vi "AWG Write Butterfly Ramps for 1Channel.vi"(6 "Secondary Pin Name":string, 7 "Main Pin Name":string, 8 "error in (no error)":errorcluster, 9 "AmpGain":dbl, 10 "Voltages":dbl[](array[numeric]), 11 "Automation Refnum in":T1) -> (0 "error out":errorcluster)   [LabVIEW 2013]
uses:
  <vilib>/NI_TestStand_SemiconductorModule/NI_TestStand_Semiconductor_Module.lvlibp/PinMap/General/SemiconductorModuleContext.ctl
  Utility/PreciseRampWaveformWithName.ctl
  Utility/PreciseRampWaveform.ctl
  <vilib>/NI_TestStand_SemiconductorModule/NI_TestStand_Semiconductor_Module.lvlibp
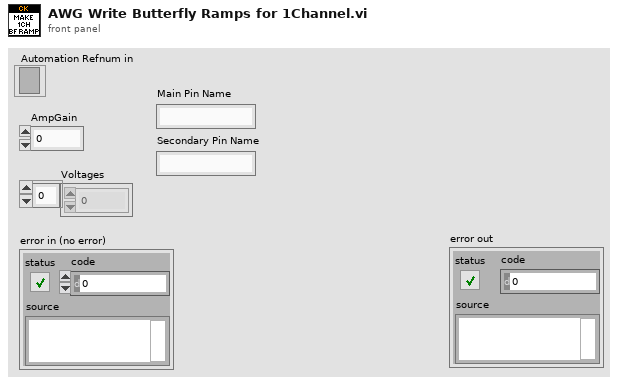
[diagram p1: front panel]
types:
  T1 = typedef "NI_TestStand_Semiconductor_Module.lvlibp/SemiconductorModuleContext.ctl" = refnum<k7>
  T2 = typedef "PreciseRampWaveformWithName.ctl" = cluster{"Name":string, "Waveform":T3}
  T3 = typedef "PreciseRampWaveform.ctl" = cluster{"Start":dbl, "End":dbl, "Time":dbl}
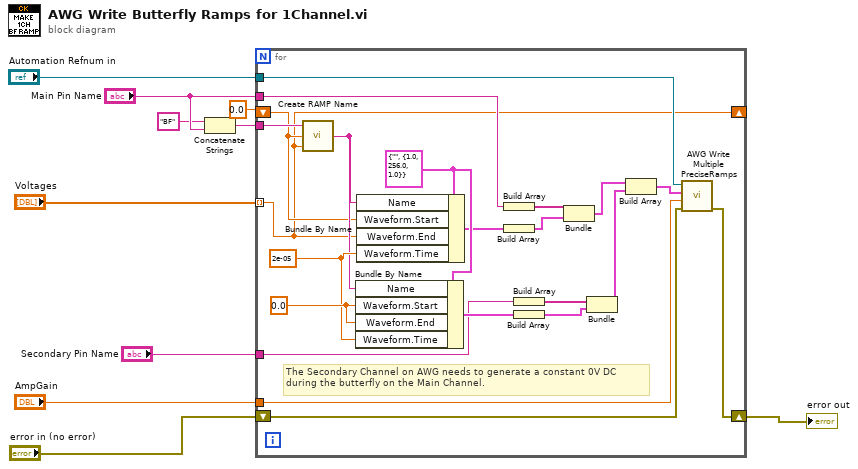
[diagram p0: block diagram]
diagram:
  n1 = Concatenate Strings("BF" ("string"), "Main Pin Name") -> (w5:string)
  n2 = for {
    tunnel: "Voltages" -> [w11] mode=indexing
    tunnel: "Automation Refnum in" -> [w32]
    tunnel: "AmpGain" -> [w30]
    shift-right: [w11] -> _
    shift-left: 0.0 ("Numeric") -> [w12]
    tunnel: "Main Pin Name" -> [w16]
    tunnel: "Secondary Pin Name" -> [w15]
    shift-right: [w14] -> w6
    shift-left: "error in (no error)" -> [w31]
    tunnel: w5 -> [w13]
    w27 = 0.0 ("Start")
    w26 = 2e-05 ("Time")
    w28 = T2 {"Name"="", "Waveform"={"Start"=1.0, "End"=256.0, "Time"=1.0}} ("Waveform In")
    # "The Secondary Channel on AWG needs to generate a constant 0V DC\nduring the butterfly on the Main Channel."
    n3 = call "Create RAMP Name.vi"("Numeric 2"=w11, "Numeric 1"=w12, "Prefix"=w13) -> ("concatenated string"=w23:string)
    n4 = Bundle By Name(cluster=w28, "Name"=w23, "Waveform.Start"=w27, "Waveform.End"=w27, "Waveform.Time"=w26) -> (w24:T2)
    n5 = Bundle By Name(cluster=w28, "Name"=w23, "Waveform.Start"=w12, "Waveform.End"=w11, "Waveform.Time"=w26) -> (w25:T2)
    n6 = Build Array(w16) -> (w18:string[])
    n7 = Build Array(w25) -> (w22:T2[])
    n8 = Build Array(w15) -> (w17:string[])
    n9 = Build Array(w24) -> (w20:T2[])
    n10 = Bundle(w18, w22) -> (w21:cluster{string[], T2[]})  [unwired: 1 in]
    n11 = Bundle(w17, w20) -> (w19:cluster{string[], T2[]})  [unwired: 1 in]
    n12 = Build Array(w21, w19) -> (w29:cluster{string[], T2[]}[])
    n13 = call "AWG Write Multiple PreciseRamps.vi"("error in (no error)"=w31, "AmpGain"=w30, "Channel Configurations"=w29, "Semiconductor Module Context"=w32) -> ("error out"=w14:errorcluster)  [unwired: 7 in]
  }
  "error out" <- w6
